vi "test.vi"(0 "object in":refnum<class "TDMSLogger_PowerScan.lvclass">, 5 "error in (no error)":errorcluster) -> (14 "object out":refnum<class "TDMSLogger_PowerScan.lvclass">, 19 "error out":errorcluster)   [LabVIEW 2023, in "TDMSLogger_PowerScan.lvclass"]
uses:
  TDMSLogger_PowerScan.lvclass
  TDMSLogger_PowerScan.lvclass/TDMSLogger_PowerScan.ctl
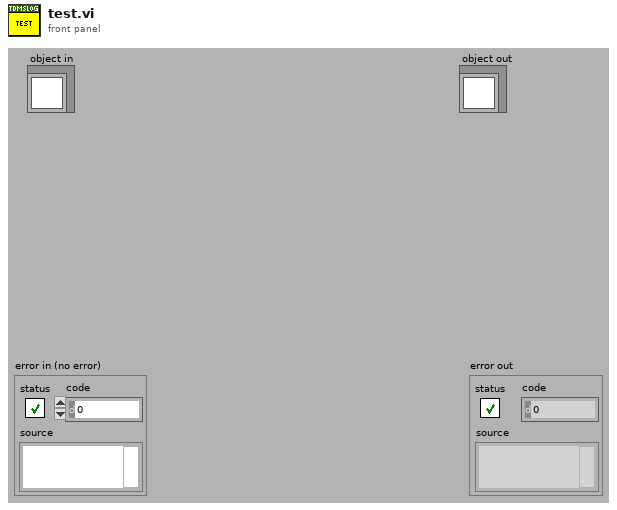
[diagram p1: front panel]
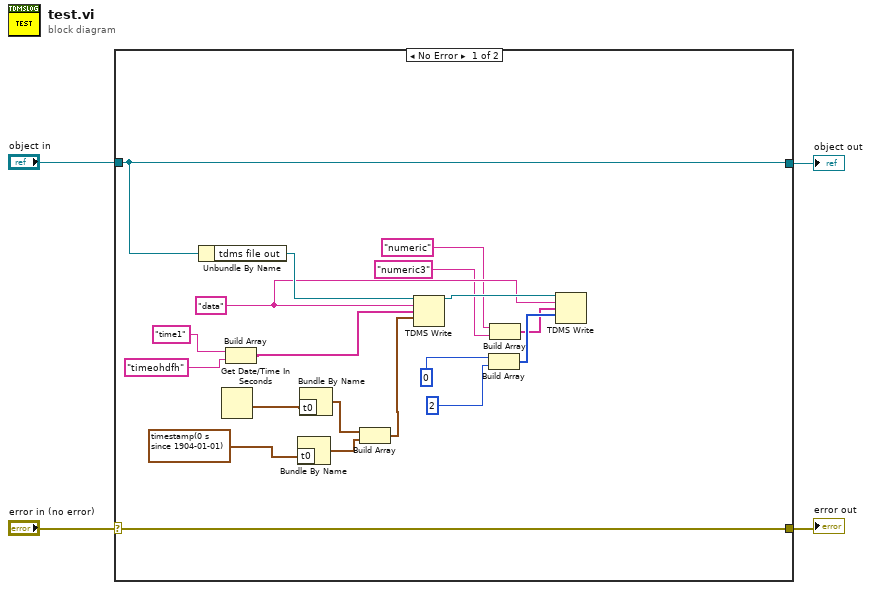
[diagram p0: block diagram]
diagram:
  n1 = case shown="No Error" "error in (no error)" {
    selector: "error in (no error)" -> [w23 w25]
    tunnel: [w23 w25] -> w3
    tunnel: [w22 w24] -> w1
    tunnel: "object in" -> [w22 w24]
    frame No Error {
      w17 = "data" ("group name in (Untitled)")
      n2 = Unbundle By Name(w22) -> ("tdms file out"=w21:refnum<k34>)
      n3 = Get Date/Time In Seconds() -> (seconds since 1Jan1904=w9:timestamp)
      n4 = Build Array("time1" ("group name in (Untitled)"), "timeohdfh" ("group name in (Untitled)")) -> (w10:string[])
      n5 = Bundle By Name("t0"=timestamp(0 s since 1904-01-01) ("element")) -> (w7:waveform(dbl))  [unwired: 1 in]
      n6 = Bundle By Name("t0"=w9) -> (w6:waveform(dbl))  [unwired: 1 in]
      n7 = Build Array(w6, w7) -> (w5:waveform(dbl)[])
      n8 = TDMS Write(0:w21, 5:w17, 7:w10, 9:w5) -> (4:w18:refnum<k34>)  [unwired: 2 in, 3 out]
      n9 = Build Array(0, 2) -> (w15:i32[])
      n10 = Build Array("numeric" ("group name in (Untitled)"), "numeric3" ("group name in (Untitled)")) -> (w13:string[])
      n11 = TDMS Write(0:w18, 5:w17, 7:w13, 9:w15) -> ()  [unwired: 2 in, 4 out]
    }
    frame Error {
    }
  }
  "error out" <- w3
  "object out" <- w1
